vi "AO Write.vi"(8 "error in (no error)":errorcluster, 10 "Analog Output":dbl format="%0.2f", 11 "FC2901 in":refnum<class "FC2901.lvclass">) -> (0 "error out":errorcluster)   [LabVIEW 2021, in "FC2901.lvclass"]
uses:
  FC2901.lvclass
  FC2901.lvclass/FC2901.ctl
  <vilib>/NathanCo/Analog-Tasks/Analog Output/Analog Output/Analog Output.lvclass
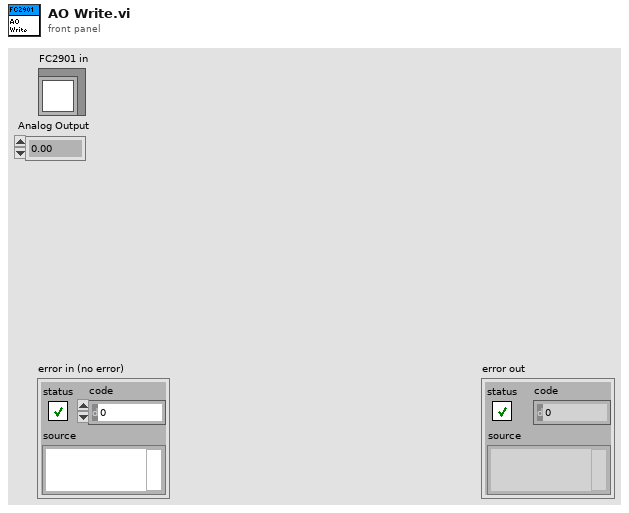
[diagram p1: front panel]
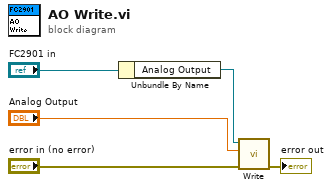
[diagram p0: block diagram]
diagram:
  n1 = Unbundle By Name("FC2901 in") -> ("Analog Output"=w3:refnum<class "Analog Output.lvclass">)
  n2 = call <vilib>:"Write.vi"("error in (no error)"="error in (no error)", "Voltage"="Analog Output", "Analog Output in"=w3) -> ("error out"=→"error out":errorcluster)  [unwired: 8 in]
